vi "Build Component Value Array.vi"(8 "error in (no error)":errorcluster, 10 "Component Name Array":string[](array[string]), 11 "Standard Display Configuration in":refnum<class "Standard Display Configuration.lvclass">) -> (0 "error out":errorcluster, 1 "Component Value Array":string[][](array[string]))   [LabVIEW 2016, in "Assert API Components.lvlib" / "Assert Display.lvlib" / "Main Display.lvlib" / "Standard Display Configuration.lvclass"]
doc: "Gets the array of component values as required by the display side of the application"
uses:
  Standard Display Configuration.lvclass
  Standard Display Configuration.lvclass/Standard Display Configuration.ctl
  Assert Display/Assert Display.lvlib
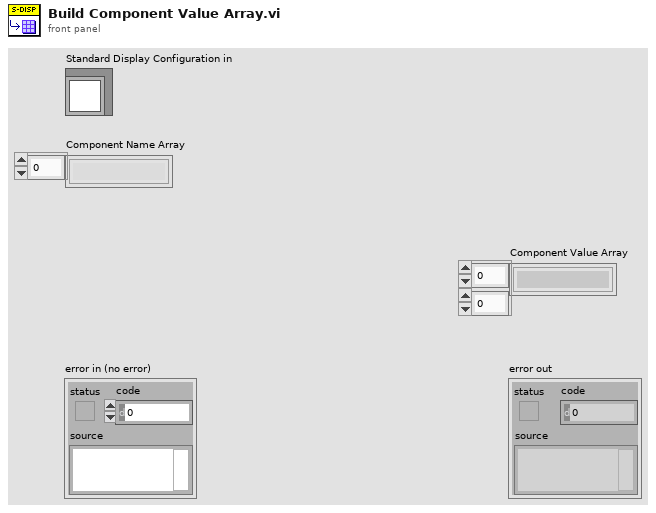
[diagram p1: front panel]
types:
  T1 = typedef "Assert API Components.lvlib/Message Data.ctl" = cluster{"Data Value":variant, "Last Update":timestamp, "Comment":string, "Evaluation String":string, "Status":bool, "Assert Name":string, "Failure Action":string, "Assert VI Name":string, "Calling VI Name":string, "Assert VI UID":i32, "Top Level VI Name":string, "VI References":T2, "Assert Build Timestamp":timestamp, "Assert Builder User Name":string, "Data Type":string}
  T2 = typedef "Assert API Components.lvlib/VI References.ctl" = cluster{"Calling VI Ref":refnum<vi>, "Assert VI Ref":refnum<vi>}
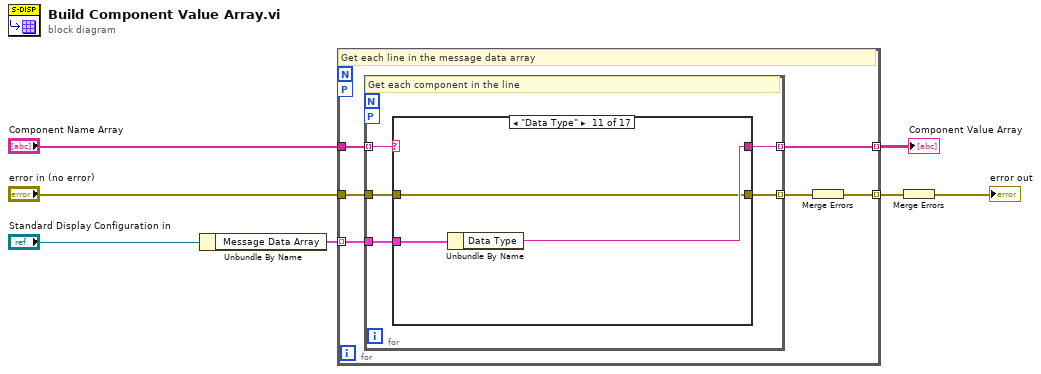
[diagram p0: block diagram]
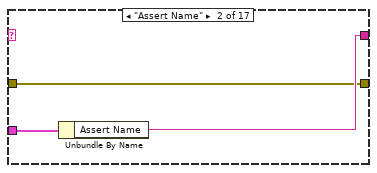
[diagram p3: hidden frame]
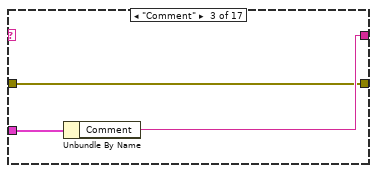
[diagram p4: hidden frame]
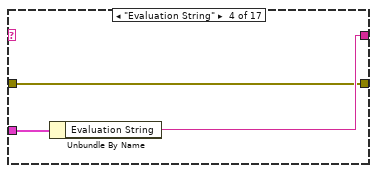
[diagram p5: hidden frame]
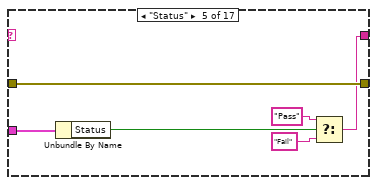
[diagram p6: hidden frame]
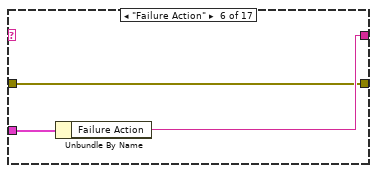
[diagram p7: hidden frame]
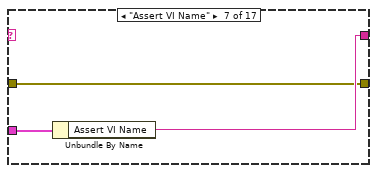
[diagram p8: hidden frame]
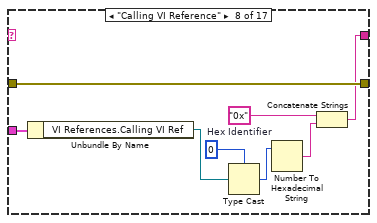
[diagram p9: hidden frame]
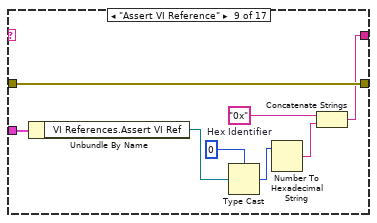
[diagram p10: hidden frame]
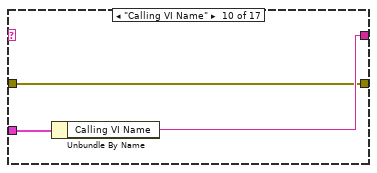
[diagram p11: hidden frame]
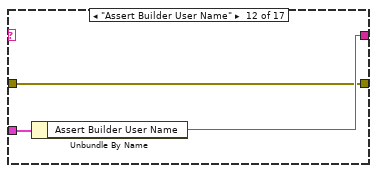
[diagram p12: hidden frame]
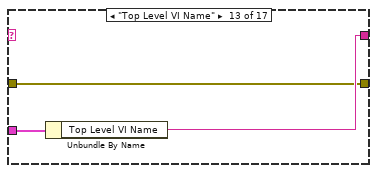
[diagram p13: hidden frame]
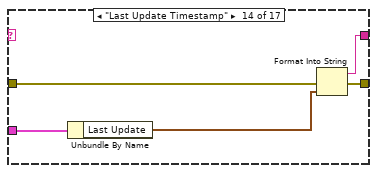
[diagram p14: hidden frame]
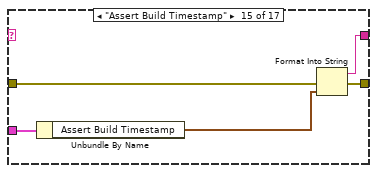
[diagram p15: hidden frame]
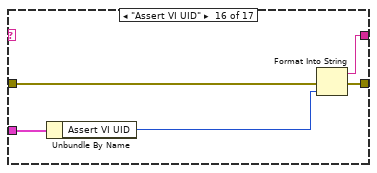
[diagram p16: hidden frame]
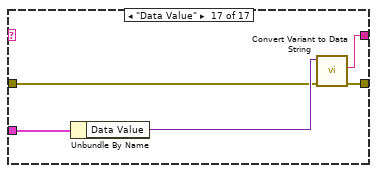
[diagram p17: hidden frame]
diagram:
  n1 = Unbundle By Name("Standard Display Configuration in") -> ("Message Data Array"=w3:T1[])
  n2 = for {
    tunnel: "Component Name Array" -> [w13]
    tunnel: w3 -> [w10] mode=indexing
    tunnel: [w9] -> w2 mode=indexing
    tunnel: "error in (no error)" -> [w12]
    tunnel: [w8] -> w5 mode=indexing
    workers-P: _ -> [_]
    # "Get each line in the message data array"
    n3 = for {
      tunnel: w13 -> [w18] mode=indexing
      tunnel: w10 -> [w15]
      tunnel: [w14] -> w9 mode=indexing
      tunnel: w12 -> [w17]
      tunnel: [w16] -> w11 mode=indexing
      workers-P: _ -> [_]
      # "Get each component in the line"
      n4 = case shown="\"Data Type\"" w18 {
        tunnel: w15 -> [_ w22 w25 w28 w34 w37 w40 w48 w56 w59 w62 w65 w68 w73 w78 w83 w88]
        tunnel: [_ w21 w24 w27 w29 w36 w39 w42 w50 w58 w61 w64 w67 w69 w74 w79 w87] -> w14
        tunnel: w17 -> [w19 w20 w23 w26 w33 w35 w38 w47 w51 w57 w60 w63 w66 w72 w77 w82 w84]
        tunnel: [w19 w20 w23 w26 w33 w35 w38 w47 w51 w57 w60 w63 w66 w71 w76 w81 w86] -> w16
        frame Default {
        }
        frame "Assert Name" {
          n5 = Unbundle By Name(w22) -> ("Assert Name"=w21:string)
        }
        frame "Comment" {
          n6 = Unbundle By Name(w25) -> ("Comment"=w24:string)
        }
        frame "Evaluation String" {
          n7 = Unbundle By Name(w28) -> ("Evaluation String"=w27:string)
        }
        frame "Status" {
          n8 = Unbundle By Name(w34) -> ("Status"=w32:bool)
          n9 = Select(t="Pass", s=w32, f="Fail") -> (s? t:f=w29:string)
        }
        frame "Failure Action" {
          n10 = Unbundle By Name(w37) -> ("Failure Action"=w36:string)
        }
        frame "Assert VI Name" {
          n11 = Unbundle By Name(w40) -> ("Assert VI Name"=w39:string)
        }
        frame "Calling VI Reference" {
          w41 = "0x"  # Hex Identifier
          n12 = Unbundle By Name(w48) -> ("VI References.Calling VI Ref"=w44:refnum<vi>)
          n13 = Type Cast(type=u32 0, x=w44) -> (*(type *) &x=w45:u32)
          n14 = Number To Hexadecimal String(2:w45) -> (0:w43:string)  [unwired: 1 in]
          n15 = Concatenate Strings(w41, w43) -> (w42:string)
        }
        frame "Assert VI Reference" {
          w49 = "0x"  # Hex Identifier
          n16 = Unbundle By Name(w56) -> ("VI References.Assert VI Ref"=w54:refnum<vi>)
          n17 = Type Cast(type=u32 0, x=w54) -> (*(type *) &x=w52:u32)
          n18 = Number To Hexadecimal String(2:w52) -> (0:w53:string)  [unwired: 1 in]
          n19 = Concatenate Strings(w49, w53) -> (w50:string)
        }
        frame "Calling VI Name" {
          n20 = Unbundle By Name(w59) -> ("Calling VI Name"=w58:string)
        }
        frame "Data Type" {
          n21 = Unbundle By Name(w62) -> ("Data Type"=w61:string)
        }
        frame "Assert Builder User Name" {
          n22 = Unbundle By Name(w65) -> ("Assert Builder User Name"=w64:string)
        }
        frame "Top Level VI Name" {
          n23 = Unbundle By Name(w68) -> ("Top Level VI Name"=w67:string)
        }
        frame "Last Update Timestamp" {
          n24 = Unbundle By Name(w73) -> ("Last Update"=w70:timestamp)
          n25 = Format Into String(error in=w72, w70) -> (resulting string=w69:string, error out=w71:errorcluster)  [unwired: 2 in]
        }
        frame "Assert Build Timestamp" {
          n26 = Unbundle By Name(w78) -> ("Assert Build Timestamp"=w75:timestamp)
          n27 = Format Into String(error in=w77, w75) -> (resulting string=w74:string, error out=w76:errorcluster)  [unwired: 2 in]
        }
        frame "Assert VI UID" {
          n28 = Unbundle By Name(w83) -> ("Assert VI UID"=w80:i32)
          n29 = Format Into String(error in=w82, w80) -> (resulting string=w79:string, error out=w81:errorcluster)  [unwired: 2 in]
        }
        frame "Data Value" {
          n30 = Unbundle By Name(w88) -> ("Data Value"=w85:variant)
          n31 = call "Convert Variant to Data String.vi"("error in (no error)"=w84, "Data Value"=w85) -> ("error out"=w86:errorcluster, "Data Value String"=w87:string)  [unwired: 8 in]
        }
      }
    }
    n32 = Merge Errors(w11) -> (w8:errorcluster)
  }
  "Component Value Array" <- w2
  n33 = Merge Errors(w5) -> (→"error out":errorcluster)
